vi "Thermopower-v2-SMU1sameasSMU2.vi"(0 "Gate Start":dbl format="%#_13g", 1 "hold time (sec)":dbl=10.0 format="%#_13g", 2 "Gate step - extra milliseconds to wait":u32=20000, 4 "N Gate Intervals":i32=7, 5 "Gate Step":dbl=-6.0, 6 "N Heater Intervals":i32=7, 7 "Heater Step":dbl=3.3) -> ()   [LabVIEW 2016]
uses:
  <vilib>/Utility/file.llb/Write To Spreadsheet File (DBL).vi
  <vilib>/Utility/file.llb/Read From Spreadsheet File (DBL).vi
  Driver/New driver/Agilent 415X Series.lvlib
panel:
  out "Voltage across heater (VSU 1 and SMU4) 2":dbl[][](graph)
  out "error out 2":errorcluster
  out "Gate Voltage (SMU 3) 2":dbl[](graph)
  out "Thermal Voltage (SMU2), SMU1 is Common 2":dbl[](graph)
  out "SPA VISA resource name 2":refnum<visa-resource-name>
  out "Voltage across heater (VSU 1 and SMU4)":dbl[][](graph)
  out "Gate Voltage (SMU 3)":dbl[](graph)
  out "Thermal Voltage (SMU2), SMU1 is Common":dbl[](graph)
  in  "SPA VISA resource name":refnum<visa-resource-name>="GPIB0::14::INSTR"
  in  "error in (no error)":errorcluster
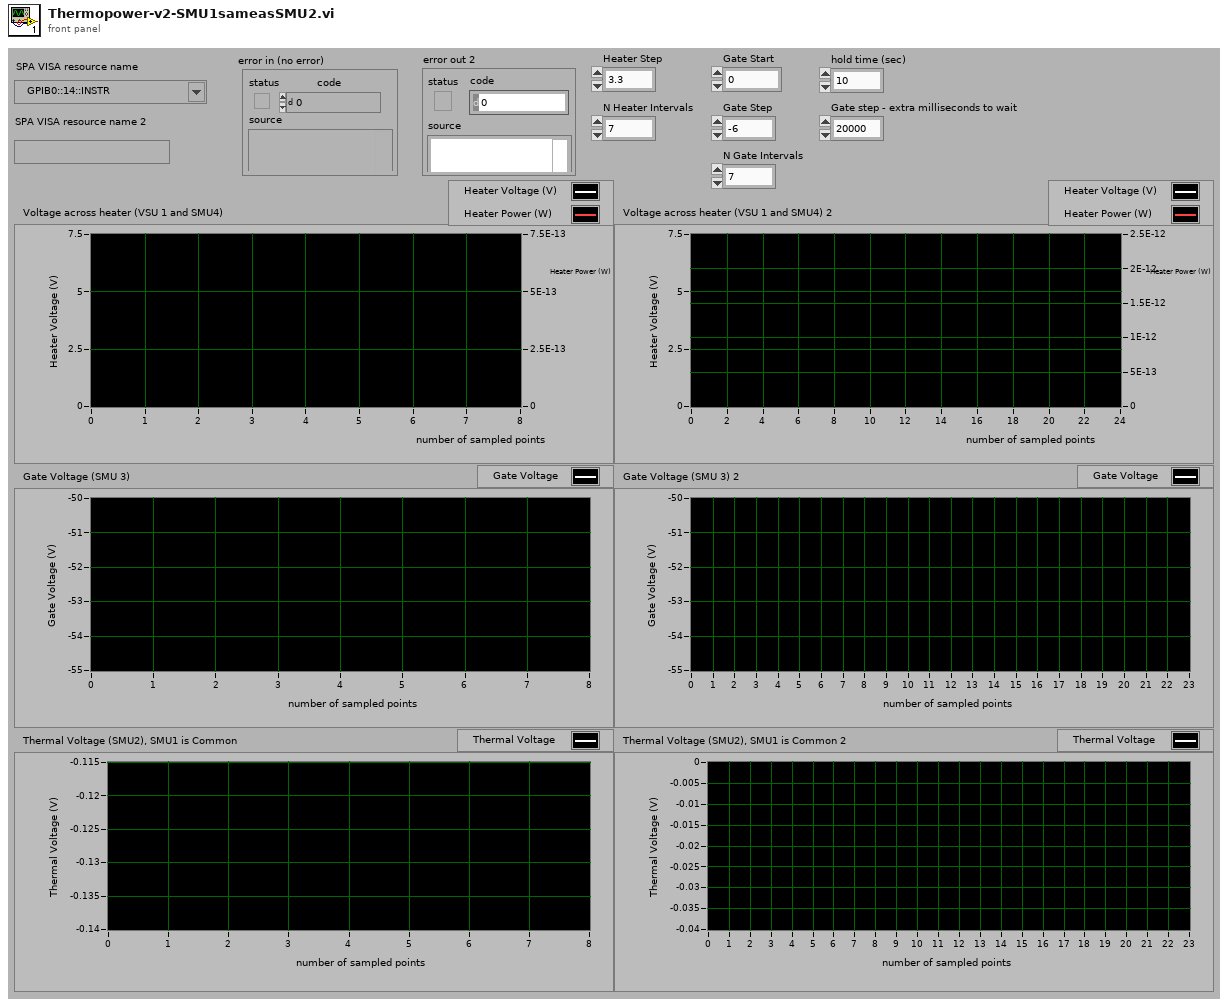
[diagram p1: front panel]
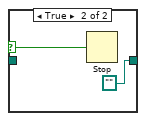
[diagram p3: hidden frame]
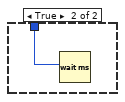
[diagram p4: hidden frame]
diagram:
  # "calculate end gate voltage"
  n1 = flat-sequence {
    tunnel: "error in (no error)" -> [w55]
    tunnel: "SPA VISA resource name" -> [w54]
    tunnel: [w53] -> w49
    tunnel: [w52] -> w48
    tunnel: w49 -> [w62]
    tunnel: w48 -> [w61]
    tunnel: [w58] -> w47
    tunnel: [w57] -> w46
    tunnel: w47 -> [w70]
    tunnel: w46 -> [w69]
    tunnel: [w68] -> w45
    tunnel: [w67] -> w44
    tunnel: w45 -> [w81]
    tunnel: w44 -> [w80]
    tunnel: [w79] -> w43
    tunnel: [w78] -> w42
    tunnel: w43 -> [w92]
    tunnel: w42 -> [w91]
    tunnel: [w90] -> w41
    tunnel: [w89] -> w39
    tunnel: w41 -> [w97]
    tunnel: [w98] -> w40
    tunnel: w39 -> [w96]
    tunnel: [w99] -> w38
    tunnel: w40 -> [w114]
    tunnel: w38 -> [w116]
    tunnel: [w115] -> w31
    tunnel: [w113] -> w30
    tunnel: w31 -> [w134]
    tunnel: w30 -> [w135]
    tunnel: [w119] -> w9
    tunnel: [w118] -> w7
    tunnel: w9 -> [w139]
    tunnel: [w138] -> w8
    tunnel: w7 -> [w140]
    tunnel: [w137] -> w6
    tunnel: [w144] -> w37
    tunnel: [w147] -> w36
    tunnel: [w146] -> w1
    tunnel: w8 -> [w144]
    tunnel: w6 -> [w145]
    frame #0 {
      n2 = call "Initialize.vi"("error in (no error)"=w55, "reset"=TRUE, "VISA resource name"=w54) -> ("error out"=w52:errorcluster, "VISA resource name out"=w53:refnum<visa-resource-name>)  [unwired: 2 in, 5 out]
    }
    frame #1 {
      n3 = call "Select-Meas. Mode.vi"("clear all channels"=TRUE, "error in (no error)"=w61, "measurement mode"=TRUE, "VISA resource name"=w62) -> ("error out"=w57:errorcluster, "VISA resource name out"=w58:refnum<visa-resource-name>)  [unwired: 1 in, 5 out]
    }
    frame #2 {
      w65 = 0 items=["0  ", "10K Ohms  ", "100K Ohms  ", "1M Ohms  "] ("series resistance *")
      w66 = 1 items=["V  ", "I  ", "  common  "] ("mode")
      w71 = 0 items=["SMU1  ", "SMU2  ", "SMU3  ", "SMU4  ", "SMU5  ", "SMU6  "] ("unit to configure")
      # "SMU1 configured to be common"
      n4 = call "Config-Chan-SMU-Sampling.vi"("VISA resource name in"=w70, "function"=TRUE, "series resistance *"=w65, "unit to configure"=w71, "V name (max 6 chars)"="Vgnd", "standby"=TRUE, "error in (no error)"=w69, "mode"=w66, "I name (max 6 chars)"="Ignd") -> ("VISA resource name out"=w68:refnum<visa-resource-name>, "error out"=w67:errorcluster)  [unwired: 5 out]
    }
    frame #3 {
      w75 = 0 items=["0  ", "10K Ohms  ", "100K Ohms  ", "1M Ohms  "] ("series resistance *")
      w77 = 1 items=["V  ", "I  ", "  common  "] ("mode")
      w82 = 1 items=["SMU1  ", "SMU2  ", "SMU3  ", "SMU4  ", "SMU5  ", "SMU6  "] ("unit to configure")
      # "SMU2 configured to source current (to be set to zero) \nand measure the thermal voltage"
      n5 = call "Config-Chan-SMU-Sampling.vi"("VISA resource name in"=w81, "function"=TRUE, "series resistance *"=w75, "unit to configure"=w82, "V name (max 6 chars)"="Vth", "standby"=TRUE, "error in (no error)"=w80, "mode"=w77, "I name (max 6 chars)"="Ith") -> ("VISA resource name out"=w79:refnum<visa-resource-name>, "error out"=w78:errorcluster)  [unwired: 5 out]
    }
    frame #4 {
      w86 = 0 items=["0  ", "10K Ohms  ", "100K Ohms  ", "1M Ohms  "] ("series resistance *")
      w88 = 0 items=["V  ", "I  ", "  common  "] ("mode")
      w93 = 2 items=["SMU1  ", "SMU2  ", "SMU3  ", "SMU4  ", "SMU5  ", "SMU6  "] ("unit to configure")
      # "SMU3 configured to source a gate voltage"
      n6 = call "Config-Chan-SMU-Sampling.vi"("VISA resource name in"=w92, "function"=TRUE, "series resistance *"=w86, "unit to configure"=w93, "V name (max 6 chars)"="Vg", "standby"=TRUE, "error in (no error)"=w91, "mode"=w88, "I name (max 6 chars)"="Ig") -> ("VISA resource name out"=w90:refnum<visa-resource-name>, "error out"=w89:errorcluster)  [unwired: 5 out]
    }
    frame #5 {
      w101 = 0 items=["0  ", "10K Ohms  ", "100K Ohms  ", "1M Ohms  "] ("series resistance *")
      w103 = 2 items=["V  ", "I  ", "  common  "] ("mode")
      w104 = 3 items=["SMU1  ", "SMU2  ", "SMU3  ", "SMU4  ", "SMU5  ", "SMU6  "] ("unit to configure")
      # "SMU4 configured to heater ground"
      n7 = call "Config-Chan-SMU-Sampling.vi"("VISA resource name in"=w97, "function"=TRUE, "series resistance *"=w101, "unit to configure"=w104, "V name (max 6 chars)"="Vhgnd", "standby"=TRUE, "error in (no error)"=w96, "mode"=w103, "I name (max 6 chars)"="Ihgnd") -> ("VISA resource name out"=w98:refnum<visa-resource-name>, "error out"=w99:errorcluster)  [unwired: 5 out]
    }
    frame #6 {
      # "VSU1 configured to source a voltage accross a heater"
      n8 = call "Config-Chan-VSUs-Sampling.vi"("VISA session"=w114, "VSU1 function"=TRUE, "VSU2 standby"=TRUE, "VSU1 standby"=FALSE, "VSU1 V name \n(max 6 chars)"="VSU1" ("V name (max 6 chars)"), "VSU2 V name \n(max 6 chars)"="VSU2" ("V name (max 6 chars)"), "error in (no error)"=w116, "VSU2 function"=FALSE) -> ("VISA resource name out"=w113:refnum<visa-resource-name>, "error out"=w115:errorcluster)  [unwired: 6 out]
    }
    frame #7 {
      n9 = VISA Write(VISA resource name=w135, write buffer=":PAGE:MEAS:MSET:SMU1:RANG:MODE FIX", error in (no error)=w134) -> (VISA resource name out=w133:refnum<visa-resource-name>, error out=w130:errorcluster)  [unwired: 1 out]
      n10 = VISA Write(VISA resource name=w133, write buffer=":PAGE:MEAS:MSET:SMU1:RANG 2", error in (no error)=w130) -> (VISA resource name out=w132:refnum<visa-resource-name>, error out=w129:errorcluster)  [unwired: 1 out]
      n11 = VISA Write(VISA resource name=w132, write buffer=":PAGE:MEAS:MSET:SMU2:RANG:MODE FIX", error in (no error)=w129) -> (VISA resource name out=w131:refnum<visa-resource-name>, error out=w128:errorcluster)  [unwired: 1 out]
      n12 = VISA Write(VISA resource name=w131, write buffer=":PAGE:MEAS:MSET:SMU2:RANG 2", error in (no error)=w128) -> (VISA resource name out=w123:refnum<visa-resource-name>, error out=w122:errorcluster)  [unwired: 1 out]
      n13 = VISA Write(VISA resource name=w123, write buffer=":PAGE:MEAS:MSET:ITIM LONG", error in (no error)=w122) -> (VISA resource name out=w121:refnum<visa-resource-name>, error out=w120:errorcluster)  [unwired: 1 out]
      n14 = VISA Write(VISA resource name=w121, write buffer=":PAGE:MEAS:MSET:ITIM:LONG 10", error in (no error)=w120) -> (VISA resource name out=w119:refnum<visa-resource-name>, error out=w118:errorcluster)  [unwired: 1 out]
    }
    frame #8 {
      w142 = u16 0 items=["SMU 1", "SMU2", "SMU3", "SMU4", "SMU5", "SMU6", "VSU1", "VSU2"] ("unit (SMU1:0)")
      n15 = call "Config-Sampling-Const-Source.vi"("compliance (SMUs only)"=0.0001, "error in (no error)"=w140, "source (V or A)"=0.0, "unit (SMU1:0)"=w142, "VISA session"=w139) -> ("error out"=w137:errorcluster, "VISA resource name out"=w138:refnum<visa-resource-name>)  [unwired: 5 out]
    }
    frame #9 {
      w146 = 0.0 ("source (V or A)")
      w148 = u16 1 items=["SMU 1", "SMU2", "SMU3", "SMU4", "SMU5", "SMU6", "VSU1", "VSU2"] ("unit (SMU1:0)")
      n16 = call "Config-Sampling-Const-Source.vi"("compliance (SMUs only)"=0.0001, "error in (no error)"=w145, "source (V or A)"=w146, "unit (SMU1:0)"=w148, "VISA session"=w144) -> ("error out"=w147:errorcluster)  [unwired: 6 out]
    }
  }
  n17 = Subtract(x="N Gate Intervals", y=1) -> (x-y=w19:i32)
  n18 = Multiply(x=w19, y="Gate Step") -> (x*y=w17:dbl)
  n19 = Add(x=w17, y="Gate Start") -> (x+y=w16:dbl)
  n20 = call "File Dialog"("start path"=path "C:/users old/khk30", "pattern (all files)"="*.txt") -> ("selected path"=w34:path, "cancelled"=w33:bool)  [unwired: 10 in, 2 out]
  n21 = case shown="False" w33 {
    selector: w33 -> [_ w152]
    tunnel: w34 -> [w150 _]
    tunnel: [w150 path ""] -> w23
    frame False {
    }
    frame True {
      n22 = Stop(stop? (T)=w152) -> ()
    }
  }
  n23 = for {
    N: "N Gate Intervals" -> [_]
    tunnel: w23 -> [w164]
    tunnel: w37 -> [w163]
    tunnel: w36 -> [w162]
    tunnel: [w160] -> w27
    tunnel: [w159] -> w26
    tunnel: "N Heater Intervals" -> [w158]
    tunnel: "Gate Step" -> [w157]
    tunnel: "Gate Start" -> [w156]
    tunnel: "Heater Step" -> [w155]
    tunnel: "Gate step - extra milliseconds to wait" -> [w154]
    tunnel: [w153] -> w12 mode=indexing
    i -> [w161]
    n24 = flat-sequence {
      tunnel: w161 -> [w321]
      tunnel: [w326] -> w166
      tunnel: [w325] -> w165
      tunnel: w163 -> [w324]
      tunnel: w162 -> [w323]
      tunnel: w157 -> [w318]
      tunnel: w156 -> [w317]
      frame #0 {
        w327 = u16 2 items=["SMU 1", "SMU2", "SMU3", "SMU4", "SMU5", "SMU6", "VSU1", "VSU2"] ("unit (SMU1:0)")
        n25 = Multiply(x=w318, y=w321) -> (x*y=w320:dbl)
        n26 = Add(x=w317, y=w320) -> (x+y=w319:dbl)
        n27 = call "Config-Sampling-Const-Source.vi"("compliance (SMUs only)"=0.001, "error in (no error)"=w323, "source (V or A)"=w319, "unit (SMU1:0)"=w327, "VISA session"=w324) -> ("error out"=w325:errorcluster, "VISA resource name out"=w326:refnum<visa-resource-name>)  [unwired: 5 out]
      }
    }
    n28 = for {
      N: w158 -> [_]
      tunnel: w166 -> [w185]
      tunnel: w165 -> [w184]
      tunnel: w164 -> [w183]
      tunnel: w161 -> [w176]
      tunnel: [w171] -> w160
      tunnel: [w170] -> w159
      tunnel: w155 -> [w169]
      tunnel: w154 -> [w168]
      tunnel: [w167] -> w153 mode=indexing
      i -> [w186]
      n29 = flat-sequence {
        tunnel: [w203] -> w196
        tunnel: [w202] -> w195
        tunnel: w186 -> [w198]
        tunnel: w185 -> [w201]
        tunnel: w184 -> [w200]
        tunnel: [w198] -> w177
        tunnel: w169 -> [w197]
        tunnel: w196 -> [w213]
        tunnel: w195 -> [w211]
        tunnel: [w212] -> w194
        tunnel: [w211] -> w193
        tunnel: w177 -> [w207]
        tunnel: w176 -> [w206]
        tunnel: w168 -> [w205]
        tunnel: w194 -> [w220]
        tunnel: w193 -> [w219]
        tunnel: [w218] -> w192
        tunnel: [w217] -> w191
        tunnel: ["hold time (sec)"] -> w167
        tunnel: w192 -> [w230]
        tunnel: w191 -> [w229]
        tunnel: [w228] -> w190
        tunnel: [w227] -> w189
        tunnel: w190 -> [w236]
        tunnel: w189 -> [w235]
        tunnel: [w234] -> w188
        tunnel: [w233] -> w187
        tunnel: w188 -> [w260]
        tunnel: w187 -> [w259]
        tunnel: w183 -> [w261]
        tunnel: [w261] -> w182
        tunnel: [w261] -> w181
        tunnel: [w243] -> w179
        tunnel: [w244] -> w171
        tunnel: w182 -> [w288]
        tunnel: [w286] -> w175
        tunnel: w181 -> [w286]
        tunnel: w179 -> [w283]
        tunnel: [w283] -> w173
        tunnel: w175 -> [w292]
        tunnel: [w292] -> w174
        tunnel: w173 -> [w293]
        tunnel: [w293] -> w172
        tunnel: w174 -> [w298]
        tunnel: [w298] -> w180
        tunnel: w172 -> [w294]
        tunnel: [w294] -> w178
        tunnel: w180 -> [w312]
        tunnel: w178 -> [w303]
        tunnel: [w303] -> w170
        frame #0 {
          w204 = u16 6 items=["SMU 1", "SMU2", "SMU3", "SMU4", "SMU5", "SMU6", "VSU1", "VSU2"] ("unit (SMU1:0)")
          n30 = Multiply(x=w197, y=w198) -> (x*y=w199:dbl)
          n31 = call "Config-Sampling-Const-Source.vi"("error in (no error)"=w200, "source (V or A)"=w199, "unit (SMU1:0)"=w204, "VISA session"=w201) -> ("error out"=w203:errorcluster, "VISA resource name out"=w202:refnum<visa-resource-name>)  [unwired: 1 in, 5 out]
        }
        frame #1 {
          n32 = Equal To 0?(x=w207) -> (x = 0?=w208:bool)
          n33 = Greater Than 0?(x=w206) -> (x > 0?=w209:bool)
          n34 = And(x=w208, y=w209) -> (x .and. y?=w210:bool)
          n35 = call "Config-Display-List.vi"("error in (no error)"=w213, "list (max 8 elements)"=string[] ["Vth", "Ith", "VSU1", "Ihgnd", "Vg", "Ig", "Ignd", "Vgnd"], "VISA session"=w211) -> ("error out"=w212:errorcluster)  [unwired: 1 in, 7 out]
          n36 = case shown="False" w210 {
            tunnel: w205 -> [_ w215]
            frame False {
            }
            frame True {
              n37 = Wait (ms)(milliseconds to wait=w215) -> ()  [unwired: 1 out]
            }
          }
        }
        frame #2 {
          w221 = 100.0  # sampling time limit
          w222 = 0 items=["linear", "log 10", "log 25", "log 50", "thinned out"] ("mode (linear: 0)")
          w223 = 0 items=["auto (linear only)", "no limit", "set limit "] ("sampling time\n(linear/thinned-out only)")
          w224 = 0.1  # initial interval (sec)
          w225 = 10  # num. of events
          w226 = 1  # number of samples
          n38 = call "Config-Sampling-Parameters.vi"("VISA session"=w219, "mode (linear: 0)"=w222, "initial interval (sec)"=w224, "sampling time\n(linear/thinned-out only)"=w223, "number of samples"=w226, "error in (no error)"=w220, "sampling time limit"=w221, "num. of events"=w225, "hold time (sec)"="hold time (sec)") -> ("VISA resource name out"=w217:refnum<visa-resource-name>, "error out"=w218:errorcluster)  [unwired: 7 in, 10 out]
        }
        frame #3 {
          w232 = 2 items=["short  ", "medium  ", "long  "] ("integration time")
          n39 = call "Config-Meas-Timing.vi"("# PLCs for long integration time"=1, "error in (no error)"=w230, "integration time"=w232, "VISA session"=w229) -> ("error out"=w228:errorcluster, "VISA resource name out"=w227:refnum<visa-resource-name>)  [unwired: 2 in, 4 out]
        }
        frame #4 {
          w238 = 1 items=["stop  ", "single  ", "single-append  ", "stress start  ", "continuous  ", "standby on  ", "standby off  ", "zero  "] ("function (stop:0)")
          n40 = call "Op-Start-Stop.vi"("time to wait (30000ms)"=600000, "error in (no error)"=w236, "function (stop:0)"=w238, "wait until finish"=TRUE, "VISA resource name"=w235) -> ("error out"=w234:errorcluster, "VISA resource name out"=w233:refnum<visa-resource-name>)  [unwired: 5 out]
        }
        frame #5 {
          # "Computes Heater power via P=VI"
          n41 = call "4155C DOWNLOAD variable.vi"("error in (no error)"=w260, "Variable name"="Vth", "VISA resource name in"=w259) -> ("error out"=w268:errorcluster, "Output data"=w242:dbl[], "VISA Resource Name out"=w273:refnum<visa-resource-name>)  [unwired: 2 out]
          n42 = call "4155C DOWNLOAD variable.vi"("error in (no error)"=w268, "Variable name"="Ith", "VISA resource name in"=w273) -> ("error out"=w267:errorcluster, "Output data"=w256:dbl[], "VISA Resource Name out"=w272:refnum<visa-resource-name>)  [unwired: 2 out]
          n43 = call "4155C DOWNLOAD variable.vi"("error in (no error)"=w267, "Variable name"="VSU1", "VISA resource name in"=w272) -> ("error out"=w266:errorcluster, "Output data"=w254:dbl[], "VISA Resource Name out"=w271:refnum<visa-resource-name>)  [unwired: 2 out]
          n44 = call "4155C DOWNLOAD variable.vi"("error in (no error)"=w266, "Variable name"="Ihgnd", "VISA resource name in"=w271) -> ("error out"=w265:errorcluster, "Output data"=w255:dbl[], "VISA Resource Name out"=w270:refnum<visa-resource-name>)  [unwired: 2 out]
          n45 = Multiply(x=w254, y=w255) -> (x*y=w258:dbl[])
          n46 = Absolute Value(x=w258) -> (abs(x)=w253:dbl[])
          n47 = call "4155C DOWNLOAD variable.vi"("error in (no error)"=w265, "Variable name"="Vg", "VISA resource name in"=w270) -> ("error out"=w264:errorcluster, "Output data"=w257:dbl[], "VISA Resource Name out"=w269:refnum<visa-resource-name>)  [unwired: 2 out]
          n48 = call "4155C DOWNLOAD variable.vi"("error in (no error)"=w264, "Variable name"="Ig", "VISA resource name in"=w269) -> ("error out"=w250:errorcluster, "Output data"=w249:dbl[], "VISA Resource Name out"=w252:refnum<visa-resource-name>)  [unwired: 2 out]
          n49 = call "4155C DOWNLOAD variable.vi"("error in (no error)"=w250, "Variable name"="Ignd", "VISA resource name in"=w252) -> ("error out"=w245:errorcluster, "Output data"=w248:dbl[], "VISA Resource Name out"=w246:refnum<visa-resource-name>)  [unwired: 2 out]
          n50 = call "4155C DOWNLOAD variable.vi"("error in (no error)"=w245, "Variable name"="Vgnd", "VISA resource name in"=w246) -> ("error out"=w243:errorcluster, "Output data"=w241:dbl[], "VISA Resource Name out"=w244:refnum<visa-resource-name>)  [unwired: 2 out]
          n51 = Subtract(x=w242, y=w241) -> (x-y=w240:dbl[])
          n52 = Build Array(w253, w254, w255, w242, w256, w257, w249, w248, w241, w240) -> (w263:dbl[][])
          n53 = call-poly <vilib>:"Write To Spreadsheet File.vi"("transpose? (no:F)"=TRUE, "format (%.3f)"="%.13f", "append to file? (new file:F)"=TRUE, "2D data"=w263, "file path (dialog if empty)"=w261) -> ()  [unwired: 1 in, 3 out]
        }
        frame #6 {
          # "plot the thermal voltage after reading the file"
          n54 = call-poly <vilib>:"Read From Spreadsheet File.vi"("transpose (no:F)"=TRUE, "format (%.3f)"="%.13f", "max characters/row  (no limit:0)"=0, "number of rows (all:-1)"=-1, "file path (dialog if empty)"=w288) -> ("all rows"=w285:dbl[][])  [unwired: 6 out]
          n55 = Index Array(array=w285, index (row)=9) -> (element=→"Thermal Voltage (SMU2), SMU1 is Common":dbl[])  [unwired: 1 in]
        }
        frame #7 {
        }
        frame #8 {
          # "plot the gate voltage after reading the file"
          n56 = call-poly <vilib>:"Read From Spreadsheet File.vi"("transpose (no:F)"=TRUE, "format (%.3f)"="%.13f", "max characters/row  (no limit:0)"=0, "number of rows (all:-1)"=-1, "file path (dialog if empty)"=w298) -> ("all rows"=w297:dbl[][])  [unwired: 6 out]
          n57 = Index Array(array=w297, index (row)=5) -> (element=→"Gate Voltage (SMU 3)":dbl[])  [unwired: 1 in]
        }
        frame #9 {
          # "plot the voltage across the heater and the \npower dissipated by the heater after reading the file"
          n58 = call-poly <vilib>:"Read From Spreadsheet File.vi"("transpose (no:F)"=TRUE, "format (%.3f)"="%.13f", "max characters/row  (no limit:0)"=0, "number of rows (all:-1)"=-1, "file path (dialog if empty)"=w312) -> ("all rows"=w310:dbl[][])  [unwired: 6 out]
          n59 = Index Array(array=w310, index (row)=1) -> (element=w304:dbl[])  [unwired: 1 in]
          n60 = Index Array(array=w310, index (row)=2) -> (element=w308:dbl[])  [unwired: 1 in]
          n61 = Multiply(x=w304, y=w308) -> (x*y=w307:dbl[])
          n62 = Absolute Value(x=w307) -> (abs(x)=w306:dbl[])
          n63 = Build Array(w304, w306) -> (→"Voltage across heater (VSU 1 and SMU4)":dbl[][])
        }
      }
    }
  }
  n64 = flat-sequence {
    tunnel: [w335] -> w29
    tunnel: [w334] -> w28
    tunnel: w27 -> [w329]
    tunnel: w26 -> [w328]
    tunnel: w29 -> [w346]
    tunnel: w28 -> [w345]
    tunnel: [w340] -> w11
    tunnel: [w339] -> w10
    tunnel: [w350] -> w5
    tunnel: [w351] -> w3
    tunnel: w11 -> [w353]
    tunnel: w10 -> [w352]
    tunnel: w5 -> [w367]
    tunnel: [w364] -> w4
    tunnel: w3 -> [w368]
    tunnel: [w365] -> w2
    tunnel: w1 -> [w366]
    tunnel: w4 -> [w374]
    tunnel: w2 -> [w375]
    tunnel: [w373] -> w24
    tunnel: [w372] -> w25
    tunnel: w1 -> [w371]
    frame #0 {
      w332 = 0 items=["0  ", "10K Ohms  ", "100K Ohms  ", "1M Ohms  "] ("series resistance *")
      w333 = 1 items=["V  ", "I  ", "  common  "] ("mode")
      w336 = 1 items=["SMU1  ", "SMU2  ", "SMU3  ", "SMU4  ", "SMU5  ", "SMU6  "] ("unit to configure")
      # "SMU2 configured to be common"
      n65 = call "Config-Chan-SMU-Sampling.vi"("VISA resource name in"=w329, "function"=TRUE, "series resistance *"=w332, "unit to configure"=w336, "V name (max 6 chars)"="Vgnd", "standby"=TRUE, "error in (no error)"=w328, "mode"=w333, "I name (max 6 chars)"="Ignd") -> ("VISA resource name out"=w335:refnum<visa-resource-name>, "error out"=w334:errorcluster)  [unwired: 5 out]
    }
    frame #1 {
      w342 = 0 items=["0  ", "10K Ohms  ", "100K Ohms  ", "1M Ohms  "] ("series resistance *")
      w344 = 1 items=["V  ", "I  ", "  common  "] ("mode")
      w347 = 0 items=["SMU1  ", "SMU2  ", "SMU3  ", "SMU4  ", "SMU5  ", "SMU6  "] ("unit to configure")
      # "SMU2 configured to source current (to be set to zero) \nand measure the thermal voltage"
      n66 = call "Config-Chan-SMU-Sampling.vi"("VISA resource name in"=w346, "function"=TRUE, "series resistance *"=w342, "unit to configure"=w347, "V name (max 6 chars)"="Vth", "standby"=TRUE, "error in (no error)"=w345, "mode"=w344, "I name (max 6 chars)"="Ith") -> ("VISA resource name out"=w340:refnum<visa-resource-name>, "error out"=w339:errorcluster)  [unwired: 5 out]
    }
    frame #2 {
      n67 = VISA Write(VISA resource name=w353, write buffer=":PAGE:MEAS:MSET:SMU1:RANG:MODE FIX", error in (no error)=w352) -> (VISA resource name out=w362:refnum<visa-resource-name>, error out=w359:errorcluster)  [unwired: 1 out]
      n68 = VISA Write(VISA resource name=w362, write buffer=":PAGE:MEAS:MSET:SMU1:RANG 2", error in (no error)=w359) -> (VISA resource name out=w361:refnum<visa-resource-name>, error out=w358:errorcluster)  [unwired: 1 out]
      n69 = VISA Write(VISA resource name=w361, write buffer=":PAGE:MEAS:MSET:SMU2:RANG:MODE FIX", error in (no error)=w358) -> (VISA resource name out=w360:refnum<visa-resource-name>, error out=w357:errorcluster)  [unwired: 1 out]
      n70 = VISA Write(VISA resource name=w360, write buffer=":PAGE:MEAS:MSET:SMU2:RANG 2", error in (no error)=w357) -> (VISA resource name out=w351:refnum<visa-resource-name>, error out=w350:errorcluster)  [unwired: 1 out]
    }
    frame #3 {
      w369 = u16 1 items=["SMU 1", "SMU2", "SMU3", "SMU4", "SMU5", "SMU6", "VSU1", "VSU2"] ("unit (SMU1:0)")
      n71 = call "Config-Sampling-Const-Source.vi"("compliance (SMUs only)"=0.0001, "error in (no error)"=w367, "source (V or A)"=w366, "unit (SMU1:0)"=w369, "VISA session"=w368) -> ("error out"=w364:errorcluster, "VISA resource name out"=w365:refnum<visa-resource-name>)  [unwired: 5 out]
    }
    frame #4 {
      w376 = u16 0 items=["SMU 1", "SMU2", "SMU3", "SMU4", "SMU5", "SMU6", "VSU1", "VSU2"] ("unit (SMU1:0)")
      n72 = call "Config-Sampling-Const-Source.vi"("compliance (SMUs only)"=0.0001, "error in (no error)"=w374, "source (V or A)"=w371, "unit (SMU1:0)"=w376, "VISA session"=w375) -> ("error out"=w372:errorcluster, "VISA resource name out"=w373:refnum<visa-resource-name>)  [unwired: 5 out]
    }
  }
  n73 = for {
    N: "N Gate Intervals" -> [_]
    tunnel: w23 -> [w389]
    tunnel: w24 -> [w388]
    tunnel: w25 -> [w387]
    tunnel: [w385] -> _
    tunnel: [w384] -> _
    tunnel: "N Heater Intervals" -> [w383]
    tunnel: w16 -> [w382]
    tunnel: "Gate Step" -> [w381]
    tunnel: "Heater Step" -> [w380]
    tunnel: "Gate step - extra milliseconds to wait" -> [w379]
    tunnel: w12 -> [w378] mode=indexing
    i -> [w386]
    n74 = flat-sequence {
      tunnel: w386 -> [w551]
      tunnel: [w556] -> w391
      tunnel: [w555] -> w390
      tunnel: w388 -> [w554]
      tunnel: w387 -> [w553]
      tunnel: w382 -> [w549]
      tunnel: w381 -> [w547]
      frame #0 {
        w557 = u16 2 items=["SMU 1", "SMU2", "SMU3", "SMU4", "SMU5", "SMU6", "VSU1", "VSU2"] ("unit (SMU1:0)")
        n75 = Multiply(x=w547, y=w551) -> (x*y=w548:dbl)
        n76 = Subtract(x=w549, y=w548) -> (x-y=w550:dbl)
        n77 = call "Config-Sampling-Const-Source.vi"("compliance (SMUs only)"=0.001, "error in (no error)"=w553, "source (V or A)"=w550, "unit (SMU1:0)"=w557, "VISA session"=w554) -> ("error out"=w555:errorcluster, "VISA resource name out"=w556:refnum<visa-resource-name>)  [unwired: 5 out]
      }
    }
    n78 = for {
      N: w383 -> [_]
      tunnel: w391 -> [w410]
      tunnel: w390 -> [w409]
      tunnel: w389 -> [w408]
      tunnel: w386 -> [w401]
      tunnel: [w396] -> w385
      tunnel: [w395] -> w384
      tunnel: w380 -> [w394]
      tunnel: w379 -> [w393]
      tunnel: w378 -> [w392] mode=indexing
      i -> [w411]
      n79 = flat-sequence {
        tunnel: [w428] -> w421
        tunnel: [w427] -> w420
        tunnel: w411 -> [w423]
        tunnel: w410 -> [w426]
        tunnel: w409 -> [w425]
        tunnel: [w423] -> w402
        tunnel: w394 -> [w422]
        tunnel: w421 -> [w438]
        tunnel: w420 -> [w436]
        tunnel: [w437] -> w419
        tunnel: [w436] -> w418
        tunnel: w402 -> [w432]
        tunnel: w401 -> [w431]
        tunnel: w393 -> [w430]
        tunnel: w419 -> [w445]
        tunnel: w418 -> [w444]
        tunnel: [w443] -> w417
        tunnel: [w442] -> w416
        tunnel: w392 -> [w441]
        tunnel: w417 -> [w455]
        tunnel: w416 -> [w454]
        tunnel: [w453] -> w415
        tunnel: [w452] -> w414
        tunnel: w415 -> [w461]
        tunnel: w414 -> [w460]
        tunnel: [w459] -> w413
        tunnel: [w458] -> w412
        tunnel: w413 -> [w485]
        tunnel: w412 -> [w484]
        tunnel: w408 -> [w486]
        tunnel: [w486] -> w407
        tunnel: [w486] -> w406
        tunnel: [w470] -> w404
        tunnel: [w469] -> w396
        tunnel: w407 -> [w513]
        tunnel: [w511] -> w400
        tunnel: w406 -> [w511]
        tunnel: w404 -> [w508]
        tunnel: [w508] -> w398
        tunnel: w400 -> [w517]
        tunnel: [w517] -> w399
        tunnel: w398 -> [w518]
        tunnel: [w518] -> w397
        tunnel: w399 -> [w523]
        tunnel: [w523] -> w405
        tunnel: w397 -> [w519]
        tunnel: [w519] -> w403
        tunnel: w405 -> [w542]
        tunnel: w403 -> [w528]
        tunnel: [w528] -> w395
        frame #0 {
          w429 = u16 6 items=["SMU 1", "SMU2", "SMU3", "SMU4", "SMU5", "SMU6", "VSU1", "VSU2"] ("unit (SMU1:0)")
          n80 = Multiply(x=w422, y=w423) -> (x*y=w424:dbl)
          n81 = call "Config-Sampling-Const-Source.vi"("error in (no error)"=w425, "source (V or A)"=w424, "unit (SMU1:0)"=w429, "VISA session"=w426) -> ("error out"=w428:errorcluster, "VISA resource name out"=w427:refnum<visa-resource-name>)  [unwired: 1 in, 5 out]
        }
        frame #1 {
          n82 = Equal To 0?(x=w432) -> (x = 0?=w433:bool)
          n83 = Greater Than 0?(x=w431) -> (x > 0?=w434:bool)
          n84 = And(x=w433, y=w434) -> (x .and. y?=w435:bool)
          n85 = call "Config-Display-List.vi"("error in (no error)"=w438, "list (max 8 elements)"=string[] ["Vth", "Ith", "VSU1", "Ihgnd", "Vg", "Ig", "Ignd", "Vgnd"], "VISA session"=w436) -> ("error out"=w437:errorcluster)  [unwired: 1 in, 7 out]
          n86 = case shown="True" w435 {
            tunnel: w430 -> [_ w440]
            frame False {
            }
            frame True {
              n87 = Wait (ms)(milliseconds to wait=w440) -> ()  [unwired: 1 out]
            }
          }
        }
        frame #2 {
          w446 = 100.0  # sampling time limit
          w447 = 0 items=["linear", "log 10", "log 25", "log 50", "thinned out"] ("mode (linear: 0)")
          w448 = 0 items=["auto (linear only)", "no limit", "set limit "] ("sampling time\n(linear/thinned-out only)")
          w449 = 0.1  # initial interval (sec)
          w450 = 10  # num. of events
          w451 = 1  # number of samples
          n88 = call "Config-Sampling-Parameters.vi"("VISA session"=w444, "mode (linear: 0)"=w447, "initial interval (sec)"=w449, "sampling time\n(linear/thinned-out only)"=w448, "number of samples"=w451, "error in (no error)"=w445, "sampling time limit"=w446, "num. of events"=w450, "hold time (sec)"=w441) -> ("VISA resource name out"=w442:refnum<visa-resource-name>, "error out"=w443:errorcluster)  [unwired: 7 in, 10 out]
        }
        frame #3 {
          w457 = 2 items=["short  ", "medium  ", "long  "] ("integration time")
          n89 = call "Config-Meas-Timing.vi"("# PLCs for long integration time"=1, "error in (no error)"=w455, "integration time"=w457, "VISA session"=w454) -> ("error out"=w453:errorcluster, "VISA resource name out"=w452:refnum<visa-resource-name>)  [unwired: 2 in, 4 out]
        }
        frame #4 {
          w463 = 1 items=["stop  ", "single  ", "single-append  ", "stress start  ", "continuous  ", "standby on  ", "standby off  ", "zero  "] ("function (stop:0)")
          n90 = call "Op-Start-Stop.vi"("time to wait (30000ms)"=600000, "error in (no error)"=w461, "function (stop:0)"=w463, "wait until finish"=TRUE, "VISA resource name"=w460) -> ("error out"=w459:errorcluster, "VISA resource name out"=w458:refnum<visa-resource-name>)  [unwired: 5 out]
        }
        frame #5 {
          # "Computes Heater power via P=VI"
          n91 = call "4155C DOWNLOAD variable.vi"("error in (no error)"=w485, "Variable name"="Vth", "VISA resource name in"=w484) -> ("error out"=w493:errorcluster, "Output data"=w467:dbl[], "VISA Resource Name out"=w498:refnum<visa-resource-name>)  [unwired: 2 out]
          n92 = call "4155C DOWNLOAD variable.vi"("error in (no error)"=w493, "Variable name"="Ith", "VISA resource name in"=w498) -> ("error out"=w492:errorcluster, "Output data"=w480:dbl[], "VISA Resource Name out"=w497:refnum<visa-resource-name>)  [unwired: 2 out]
          n93 = call "4155C DOWNLOAD variable.vi"("error in (no error)"=w492, "Variable name"="VSU1", "VISA resource name in"=w497) -> ("error out"=w491:errorcluster, "Output data"=w478:dbl[], "VISA Resource Name out"=w496:refnum<visa-resource-name>)  [unwired: 2 out]
          n94 = call "4155C DOWNLOAD variable.vi"("error in (no error)"=w491, "Variable name"="Ihgnd", "VISA resource name in"=w496) -> ("error out"=w490:errorcluster, "Output data"=w479:dbl[], "VISA Resource Name out"=w495:refnum<visa-resource-name>)  [unwired: 2 out]
          n95 = Multiply(x=w478, y=w479) -> (x*y=w483:dbl[])
          n96 = Absolute Value(x=w483) -> (abs(x)=w477:dbl[])
          n97 = call "4155C DOWNLOAD variable.vi"("error in (no error)"=w490, "Variable name"="Vg", "VISA resource name in"=w495) -> ("error out"=w489:errorcluster, "Output data"=w481:dbl[], "VISA Resource Name out"=w494:refnum<visa-resource-name>)  [unwired: 2 out]
          n98 = call "4155C DOWNLOAD variable.vi"("error in (no error)"=w489, "Variable name"="Ig", "VISA resource name in"=w494) -> ("error out"=w475:errorcluster, "Output data"=w482:dbl[], "VISA Resource Name out"=w476:refnum<visa-resource-name>)  [unwired: 2 out]
          n99 = call "4155C DOWNLOAD variable.vi"("error in (no error)"=w475, "Variable name"="Ignd", "VISA resource name in"=w476) -> ("error out"=w471:errorcluster, "Output data"=w474:dbl[], "VISA Resource Name out"=w472:refnum<visa-resource-name>)  [unwired: 2 out]
          n100 = call "4155C DOWNLOAD variable.vi"("error in (no error)"=w471, "Variable name"="Vgnd", "VISA resource name in"=w472) -> ("error out"=w470:errorcluster, "Output data"=w466:dbl[], "VISA Resource Name out"=w469:refnum<visa-resource-name>)  [unwired: 2 out]
          "SPA VISA resource name 2" <- w469
          n101 = Subtract(x=w467, y=w466) -> (x-y=w465:dbl[])
          n102 = Build Array(w477, w478, w479, w467, w480, w481, w482, w474, w466, w465) -> (w488:dbl[][])
          n103 = call-poly <vilib>:"Write To Spreadsheet File.vi"("transpose? (no:F)"=TRUE, "format (%.3f)"="%.13f", "append to file? (new file:F)"=TRUE, "2D data"=w488, "file path (dialog if empty)"=w486) -> ()  [unwired: 1 in, 3 out]
        }
        frame #6 {
          # "plot the thermal voltage after reading the file"
          n104 = call-poly <vilib>:"Read From Spreadsheet File.vi"("transpose (no:F)"=TRUE, "format (%.3f)"="%.13f", "max characters/row  (no limit:0)"=0, "number of rows (all:-1)"=-1, "file path (dialog if empty)"=w513) -> ("all rows"=w510:dbl[][])  [unwired: 6 out]
          n105 = Index Array(array=w510, index (row)=9) -> (element=→"Thermal Voltage (SMU2), SMU1 is Common 2":dbl[])  [unwired: 1 in]
        }
        frame #7 {
        }
        frame #8 {
          # "plot the gate voltage after reading the file"
          n106 = call-poly <vilib>:"Read From Spreadsheet File.vi"("transpose (no:F)"=TRUE, "format (%.3f)"="%.13f", "max characters/row  (no limit:0)"=0, "number of rows (all:-1)"=-1, "file path (dialog if empty)"=w523) -> ("all rows"=w522:dbl[][])  [unwired: 6 out]
          n107 = Index Array(array=w522, index (row)=5) -> (element=→"Gate Voltage (SMU 3) 2":dbl[])  [unwired: 1 in]
        }
        frame #9 {
          # "plot the voltage across the heater and the \npower dissipated by the heater after reading the file"
          n108 = call-poly <vilib>:"Read From Spreadsheet File.vi"("transpose (no:F)"=TRUE, "format (%.3f)"="%.13f", "max characters/row  (no limit:0)"=0, "number of rows (all:-1)"=-1, "file path (dialog if empty)"=w542) -> ("all rows"=w540:dbl[][])  [unwired: 6 out]
          n109 = Index Array(array=w540, index (row)=1) -> (element=w534:dbl[])  [unwired: 1 in]
          n110 = Index Array(array=w540, index (row)=2) -> (element=w538:dbl[])  [unwired: 1 in]
          n111 = property on="Voltage across heater (VSU 1 and SMU4) 2" class="WFGraph (strict)"(error in=w528, "Active Plot"=u32 0, "Plot.YScaleIdx"=u32 0 ("Plot.Y Scale Index"), "Active Plot"=u32 1, "Plot.YScaleIdx"=u32 1 ("Plot.Y Scale Index")) -> (error out=→"error out 2":errorcluster)  [unwired: 1 in, 1 out]
          n112 = Multiply(x=w534, y=w538) -> (x*y=w537:dbl[])
          n113 = Absolute Value(x=w537) -> (abs(x)=w536:dbl[])
          n114 = Build Array(w534, w536) -> (→"Voltage across heater (VSU 1 and SMU4) 2":dbl[][])
        }
      }
    }
  }
